vi "Distance Drive Checker.vi"(9 "Current Heading Target":dbl, 10 "Current Y Target":dbl, 11 "Current X Target":dbl) -> (3 "Distance Drive Done?":bool)   [LabVIEW 2014]
uses:
  Robot Global Data.vi
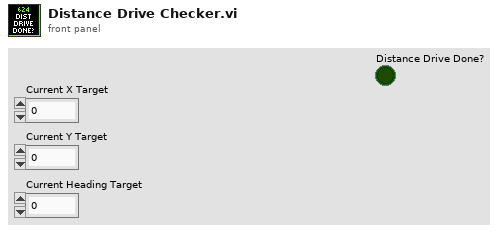
[diagram p1: front panel]
types:
  T1 = typedef "Drivetrain Status.ctl" = cluster{"Y (Throttle)":dbl, "X (Steer)":dbl, "Translation X":dbl, "Center Wheel Down":bool, "Mode":T2, "Distance Drive finished?":bool, "Y Target":dbl, "X Target":dbl, "Heading Target":dbl}
  T2 = typedef "Drivetrain Mode.ctl" = enum16{"Manual", "Gyro Steer", "Vision Steer", "Drive Distance"}
  T3 = typedef "Drivetrain Control.ctl" = cluster{"Mode":T2, "Steer":dbl, "Y":dbl, "Heading Target":dbl, "Strafe X":dbl, "Y Target":dbl, "Strafe Target":dbl}
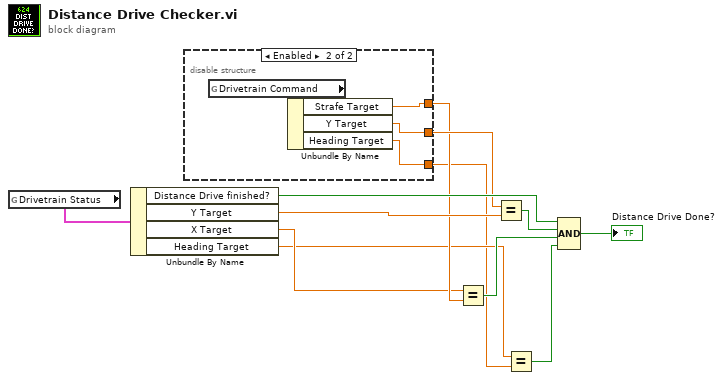
[diagram p0: block diagram]
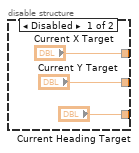
[diagram p2: hidden frame]
diagram:
  n1 = global read "Robot Global Data.vi" "Drivetrain Status"() -> (w12:T1)
  n2 = Unbundle By Name(w12) -> ("Distance Drive finished?"=w11:bool, "Y Target"=w9:dbl, "X Target"=w6:dbl, "Heading Target"=w4:dbl)
  n3 = disable-structure shown="Enabled" {
    disable-tunnel: ["Current Y Target" w17] -> w10
    disable-tunnel: ["Current X Target" w18] -> w7
    disable-tunnel: ["Current Heading Target" w16] -> w3
    frame Disabled {
    }
    frame Enabled {
      n4 = global read "Robot Global Data.vi" "Drivetrain Command"() -> (w19:T3)
      n5 = Unbundle By Name(w19) -> ("Strafe Target"=w18:dbl, "Y Target"=w17:dbl, "Heading Target"=w16:dbl)
    }
  }
  n6 = Equal?(x=w6, y=w7) -> (x = y?=w5:bool)
  n7 = Equal?(x=w10, y=w9) -> (x = y?=w8:bool)
  n8 = Equal?(x=w4, y=w3) -> (x = y?=w2:bool)
  n9 = Compound Arithmetic op=AND(w11, w8, w5, w2) -> (→"Distance Drive Done?":bool)
